vi "testValidNumber.vi"(8 "error in (no error)":errorcluster, 11 "TestCase in":refnum<class "NumberCheckerTestCase.lvclass">) -> (0 "error out":errorcluster, 3 "TestCase out":refnum<class "NumberCheckerTestCase.lvclass">)   [LabVIEW 2017, in "NumberCheckerTestCase.lvclass"]
uses:
  NumberCheckerTestCase.lvclass
  <vilib>/addons/_JKI Toolkits/VI Tester/TestCase.llb/TestCase.lvclass
  C:/Program Files (x86)/National Instruments/LabVIEW 2017/vi.lib/addons/_JKI Toolkits/VI Tester/TestCase.llb/TestCase.lvclass
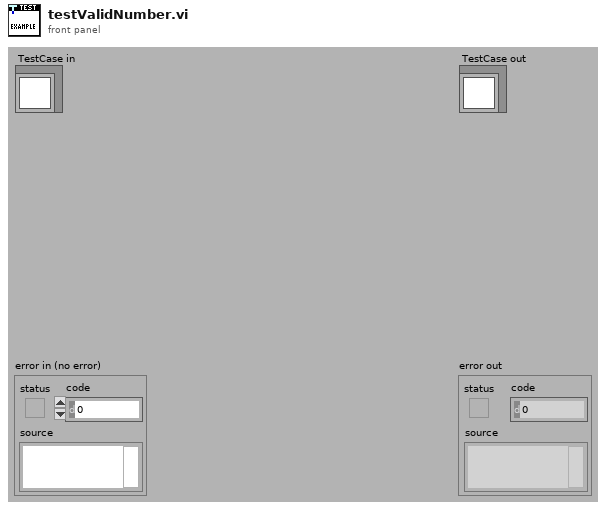
[diagram p1: front panel]
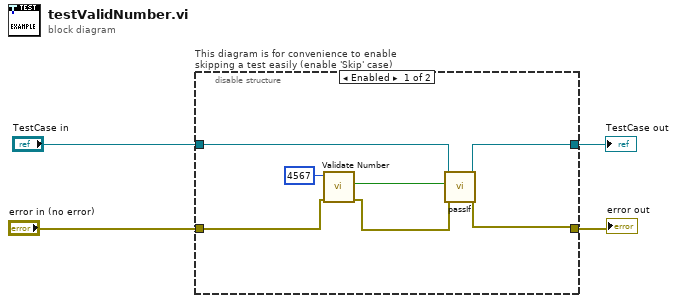
[diagram p0: block diagram]
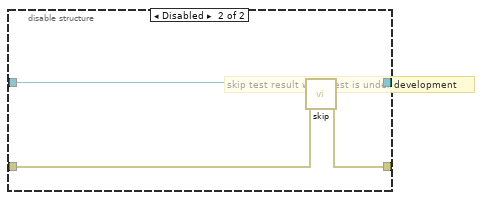
[diagram p2: hidden frame]
diagram:
  n1 = disable-structure "This diagram is for convenience to enable skipping a test easily (enable 'Skip' case)" shown="Enabled" {
    disable-tunnel: "TestCase in" -> [w11 w15]
    disable-tunnel: [w10 w13] -> w1
    disable-tunnel: [w9 w14] -> w3
    disable-tunnel: "error in (no error)" -> [w7 w12]
    frame Enabled {
      n2 = call "Validate Number.vi"("error in (no error)"=w7, "Number"=4567) -> ("error out"=w6:errorcluster, "Valid?"=w8:bool)  [unwired: 8 in]
      n3 = call-dynamic "passIf.vi"("error in (no error)"=w6, "pass"=w8, "TestCase in"=w11) -> ("error out"=w9:errorcluster, "TestCase out"=w10:refnum<class "NumberCheckerTestCase.lvclass">)  [unwired: 7 in]
    }
    frame Disabled {
      # "skip test result while test is under development"
      n4 = call <vilib>:"skip.vi"("error in (no error)"=w12, "TestCase in"=w15) -> ("error out"=w14:errorcluster, "TestCase out"=w13:refnum<class "NumberCheckerTestCase.lvclass">)  [unwired: 8 in]
    }
  }
  "error out" <- w3
  "TestCase out" <- w1
